vi "Set IRead Temperatures Multichannel.vi"(10 "IRead Temperatures Multichannel":refnum<class "IRead Temperature Multichannel.lvclass">, 11 "Thermometer Multichannel Worker in":refnum<class "Thermometer Multichannel Worker.lvclass">) -> (3 "Thermometer Multichannel Worker out":refnum<class "Thermometer Multichannel Worker.lvclass">)   [LabVIEW 2024, in "Thermometer Multichannel Worker.lvlib" / "Thermometer Multichannel Worker.lvclass"]
uses:
  Thermometer Multichannel Worker.lvclass
  Interfaces/IRead Temperature Multichannel/IRead Temperature Multichannel.lvclass
  Thermometer Multichannel Worker.lvclass/Thermometer Multichannel Worker.ctl
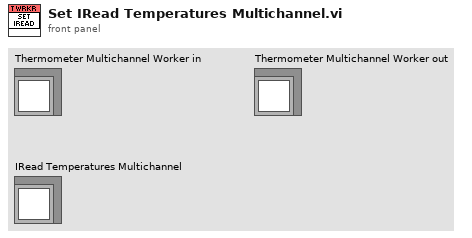
[diagram p1: front panel]
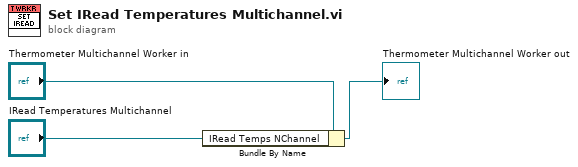
[diagram p0: block diagram]
diagram:
  n1 = Bundle By Name(cluster="Thermometer Multichannel Worker in", "IRead Temps NChannel"="IRead Temperatures Multichannel") -> (→"Thermometer Multichannel Worker out":refnum<class "Thermometer Multichannel Worker.lvclass">)
